vi "Handle Error.vi"(8 "error in (no error)":errorcluster, 11 "Recipe Process in":refnum<class "Recipe Process.lvclass">) -> (0 "error out":errorcluster, 2 "stop actor?":bool=TRUE, 3 "Recipe Process out":refnum<class "Recipe Process.lvclass">)   [LabVIEW 2022 SP3, in "Recipe Process.lvlib" / "Recipe Process.lvclass"]
doc: "(<B>Filename</B>: Actor Framework.lvlib:Actor.lvclass:Handle Error.vi)\n\nDefines how the actor handles an error that occurred while processing a message.\n\nBy default, this method does nothing except stop the actor. This method also treats error code 43 (coming from <B>error in</B>) as a sign that the actor shut down normally. In this situation, the Handle Error method does not return the error on <B>error out</B>, meaning the actor's caller will not receive it. All other error codes will be returned on <B>error out</B>.\n\nA descendant class may override this method to change this behavior."
uses:
  Recipe Process.lvclass
  Recipe Process.lvclass/Recipe Process.ctl
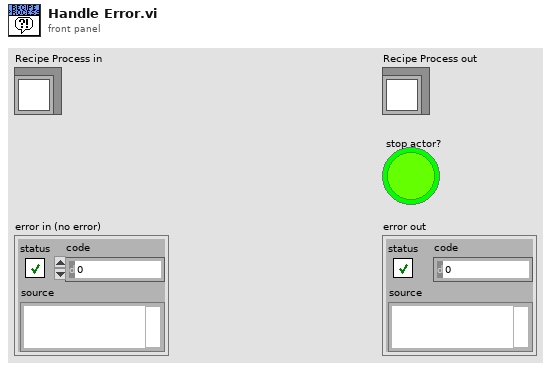
[diagram p1: front panel]
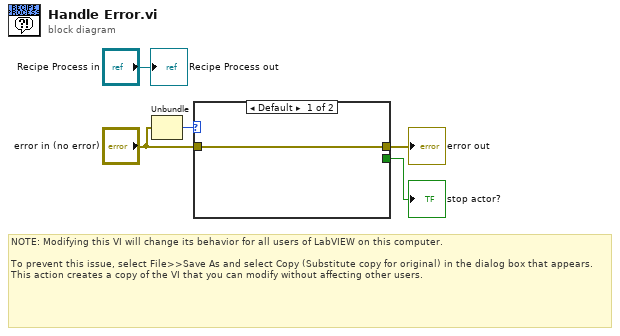
[diagram p0: block diagram]
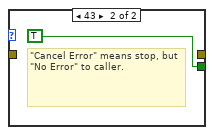
[diagram p2: hidden frame]
diagram:
  # "NOTE: Modifying this VI will change its behavior for all users of LabVIEW on this computer.\n\nTo prevent this issue, select File>>Save As and select Copy (Substitute copy for original) in the dialog box that appears. This action creates a copy of the VI that you can modify without affecting other users."
  n1 = Unbundle("error in (no error)") -> ("code"=w2:i32)  [unwired: 2 out]
  n2 = case shown="Default" w2 {
    tunnel: [w6 _] -> w5
    tunnel: "error in (no error)" -> [w6 _]
    tunnel: [_ TRUE] -> w1
    frame Default {
    }
    frame 43 {
      # "\"Cancel Error\" means stop, but \"No Error\" to caller."
    }
  }
  "error out" <- w5
  "stop actor?" <- w1
  "Recipe Process out" <- "Recipe Process in"
